vi "Average Realtime.vi"(8 "error in":errorcluster, 10 "Current Step":u32, 11 "Scan Driver.lvclass":refnum<class "Scan Driver.lvclass">) -> (0 "error out":errorcluster, 3 "Scan Driver.lvclass out":refnum<class "Scan Driver.lvclass">)   [LabVIEW 2009, in "Scan Driver.lvclass"]
uses:
  Scan Driver.lvclass
  Scan Driver.lvclass/Scan Driver.ctl
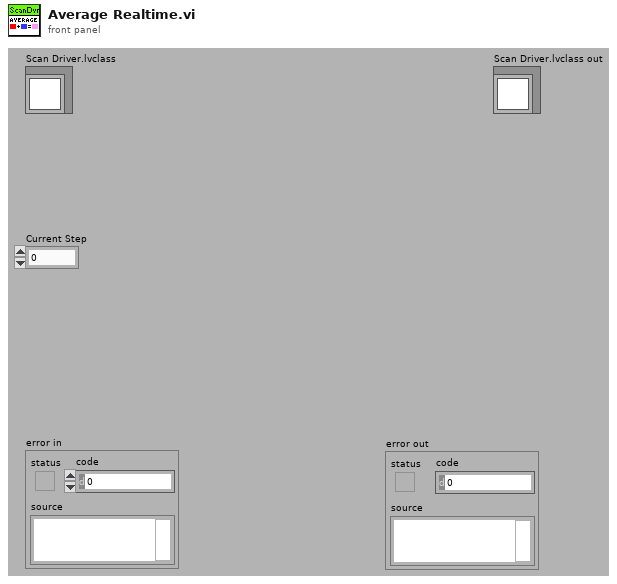
[diagram p1: front panel]
types:
  T1 = typedef "Readable.lvclass/Data Store.ctl" = T2[][]
  T2 = typedef "Readable.lvclass/Data Point.ctl" = cluster{"t":T3, "x":T4}
  T3 = typedef "Readable.lvclass/Time.ctl" = timestamp
  T4 = typedef "Readable.lvclass/X.ctl" = dbl
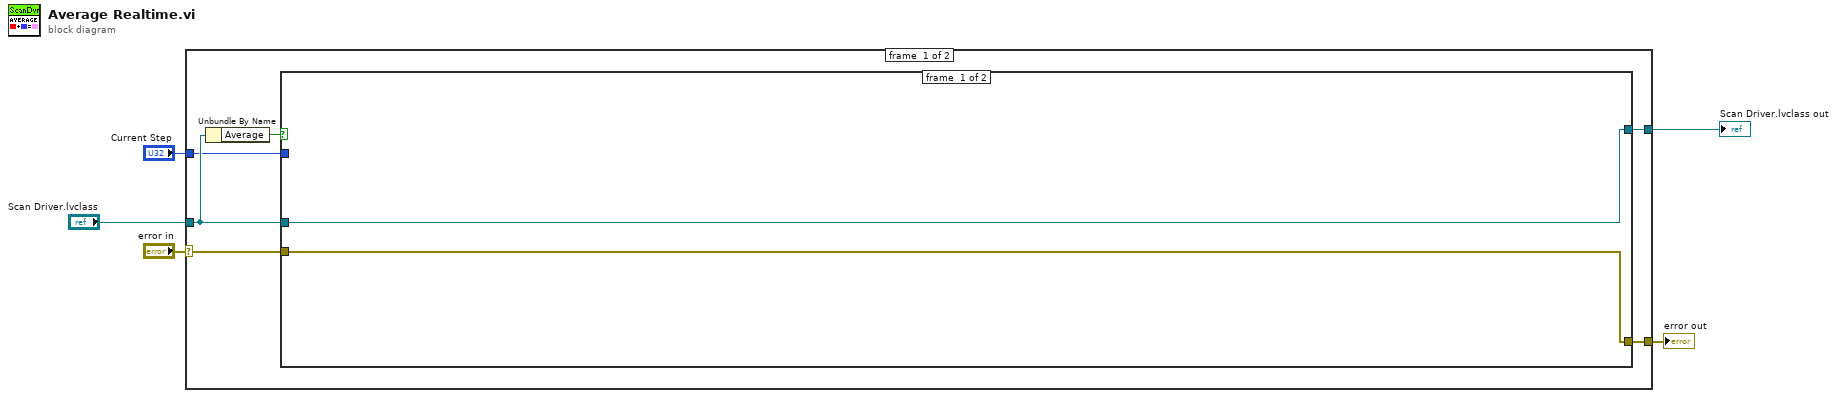
[diagram p0: block diagram]
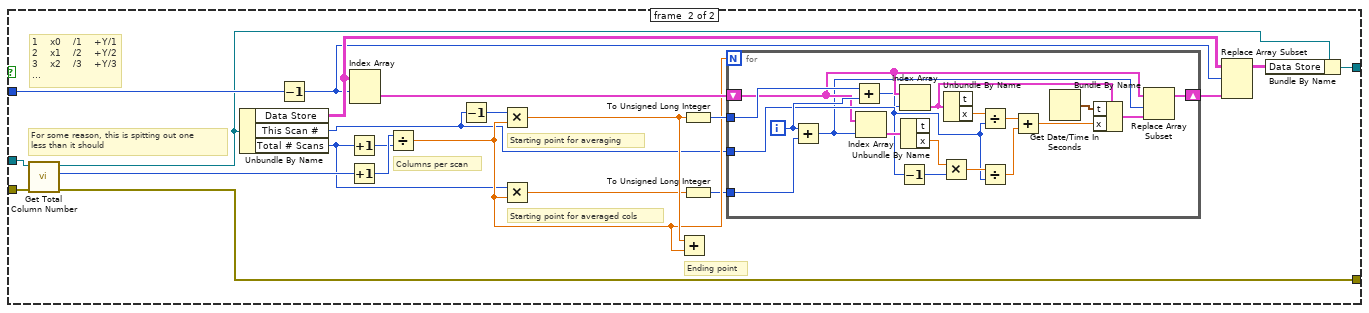
[diagram p2: hidden frame]
diagram:
  n1 = case shown="No Error" "error in" {
    selector: "error in" -> [w9 w55]
    tunnel: "Scan Driver.lvclass" -> [w11 w56]
    tunnel: [w8 w56] -> w3
    tunnel: [w7 w55] -> w2
    tunnel: "Current Step" -> [w6 _]
    frame #0 {
      n2 = Unbundle By Name(w11) -> ("Average"=w10:bool)
      n3 = case shown="True" w10 {
        tunnel: w11 -> [w13 w35]
        tunnel: w9 -> [w12 w34]
        tunnel: [w13 w32] -> w8
        tunnel: [w12 w33] -> w7
        tunnel: w6 -> [_ w31]
        frame #0 {
        }
        frame #1 {
          # "For some reason, this is spitting out one \nless than it should"
          # "1    x0    /1    +Y/1\n2    x1    /2    +Y/2\n3    x2    /3    +Y/3\n..."
          # "Starting point for averaged cols"
          # "Ending point"
          # "Starting point for averaging"
          # "Columns per scan"
          n4 = call "Get Total Column Number.vi"("error in (no error)"=w34, "Scan Driver.lvclass"=w35) -> ("error out"=w33:errorcluster, "# of Columns"=w29:i32, "Scan Driver.lvclass"=w30:refnum<class "Scan Driver.lvclass">)  [unwired: 7 in]
          n5 = Unbundle By Name(w30) -> ("Data Store"=w20:T1, "This Scan #"=w21:u32, "Total # Scans"=w16:u32)
          n6 = Decrement(x=w31) -> (x-1=w19:u32)
          n7 = Increment(x=w16) -> (x+1=w14:u32)
          n8 = Increment(x=w29) -> (x+1=w15:i32)
          n9 = Index Array(array=w20, index (row)=w19) -> (element=w27:T2[])  [unwired: 1 in]
          n10 = Divide(x=w15, y=w14) -> (x/y=w24:dbl)
          n11 = Decrement(x=w21) -> (x-1=w28:u32)
          n12 = Multiply(x=w28, y=w24) -> (x*y=w26:dbl)
          n13 = Multiply(x=w16, y=w24) -> (x*y=w23:dbl)
          n14 = Add(x=w26, y=w24) -> ()  [unwired: 1 out]
          n15 = To Unsigned Long Integer(number=w26) -> (unsigned 32bit integer=w25:u32)
          n16 = To Unsigned Long Integer(number=w23) -> (unsigned 32bit integer=w22:u32)
          n17 = for {
            N: w24 -> [_]
            tunnel: w25 -> [w54]
            tunnel: w22 -> [w52]
            tunnel: w21 -> [w45]
            shift-right: [w37] -> w17
            shift-left: w27 -> [w39]
            i -> [w53]
            n18 = Add(x=w53, y=w52) -> (x+y=w36:u32)
            n19 = Add(x=w54, y=w53) -> (x+y=w38:u32)
            n20 = Index Array(array=w39, index=w36) -> (element=w51:T2)
            n21 = Decrement(x=w45) -> (x-1=w44:u32)
            n22 = Index Array(array=w39, index=w38) -> (element=w50:T2)
            n23 = Unbundle By Name(w51) -> ("x"=w48:T4)  [unwired: 1 out]
            n24 = Multiply(x=w48, y=w44) -> (x*y=w47:T4)
            n25 = Unbundle By Name(w50) -> ("x"=w46:T4)  [unwired: 1 out]
            n26 = Divide(x=w46, y=w45) -> (x/y=w43:T4)
            n27 = Divide(x=w47, y=w45) -> (x/y=w42:T4)
            n28 = Add(x=w43, y=w42) -> (x+y=w41:T4)
            n29 = Get Date/Time In Seconds() -> (seconds since 1Jan1904=w49:timestamp)
            n30 = Bundle By Name(cluster=w50, "t"=w49, "x"=w41) -> (w40:T2)
            n31 = Replace Array Subset(array=w39, new element=w40, index=w36) -> (w37:T2[])
          }
          n32 = Replace Array Subset(array=w20, new element=w17, index (row)=w19) -> (w18:T1)  [unwired: 1 in]
          n33 = Bundle By Name(cluster=w30, "Data Store"=w18) -> (w32:refnum<class "Scan Driver.lvclass">)
        }
      }
    }
    frame #1 {
    }
  }
  "Scan Driver.lvclass out" <- w3
  "error out" <- w2
